vi "Validate_Destination_Core.vi"(8 "error in (no error)":errorcluster, 10 "Destination":refnum<class "AB_Destination.lvclass">, 11 "AB_Source_VI in":refnum<class "AB_Source_VI.lvclass">) -> (0 "error out":errorcluster, 2 "valid":bool, 3 "AB_Source_VI out":refnum<class "AB_Source_VI.lvclass">)   [LabVIEW 2020, in "AB_Source_VI.lvclass"]
uses:
  <vilib>/AppBuilder/AB_Classes/Source/VI/AB_Source_VI.lvclass
  <vilib>/AppBuilder/AB_Classes/Destination/AB_Destination.lvclass
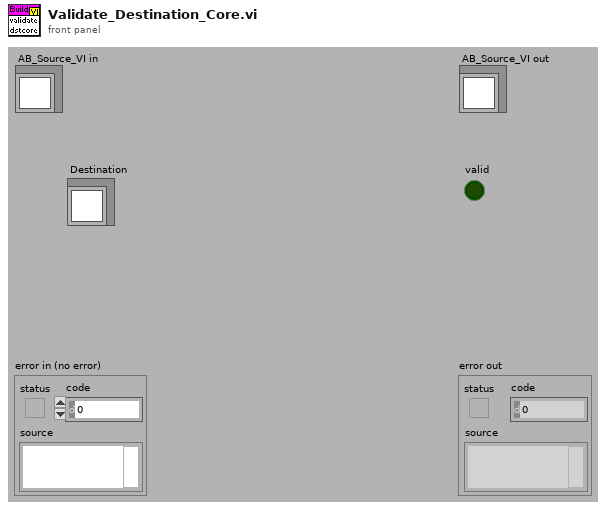
[diagram p1: front panel]
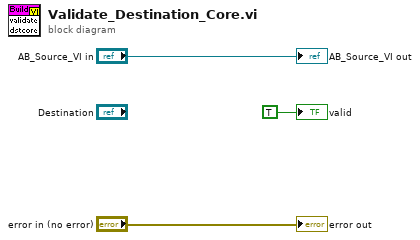
[diagram p0: block diagram]
diagram:
  "error out" <- "error in (no error)"
  "valid" <- TRUE ("valid")
  "AB_Source_VI out" <- "AB_Source_VI in"
